vi "ImageColorRgbaU32ToArray.vi"(8 "error in":errorcluster, 10 "Optional Rectangle":T2, 11 "Image Reference In":T3) -> (0 "error out":errorcluster, 2 "Pixel":T1[][](array[typedef]), 3 "Image Reference Out":T3)   [LabVIEW 2020, in "OpenLvVision_Image.lvlib" / "DataAccess.lvlib"]
doc: "Copies the pixel into an 2D array without an border."
uses:
  DataAccess.lvlib
  Management/TypeDef/Image.ctl
  TypeDef/RectangleI32.ctl
  TypeDef/RgbaU32.ctl
  TypeDef/StepSizes.ctl
  Management/Management.lvlib
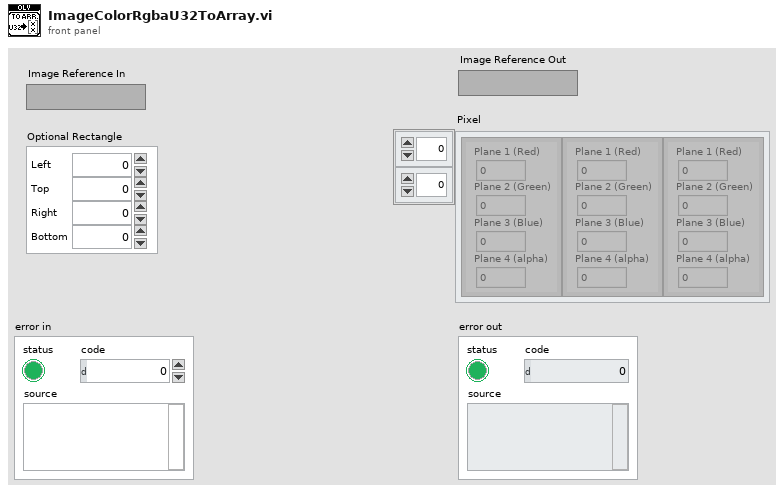
[diagram p1: front panel]
types:
  T1 = typedef "OpenLvVision_Image.lvlib/DataAccess.lvlib/RgbaU32.ctl" = cluster{"Plane 1 (Red)":u8, "Plane 2 (Green)":u8, "Plane 3 (Blue)":u8, "Plane 4 (alpha)":u8}
  T2 = typedef "OpenLvVision_Image.lvlib/DataAccess.lvlib/RectangleI32.ctl" = cluster{"Left":i32, "Top":i32, "Right":i32, "Bottom":i32}
  T3 = typedef "OpenLvVision_Image.lvlib/Management.lvlib/Image.ctl" = refnum<image>
  T4 = typedef "OpenLvVision_Image.lvlib/DataAccess.lvlib/StepSizes.ctl" = cluster{"X Step Size":u32, "Y Step Size":u32}
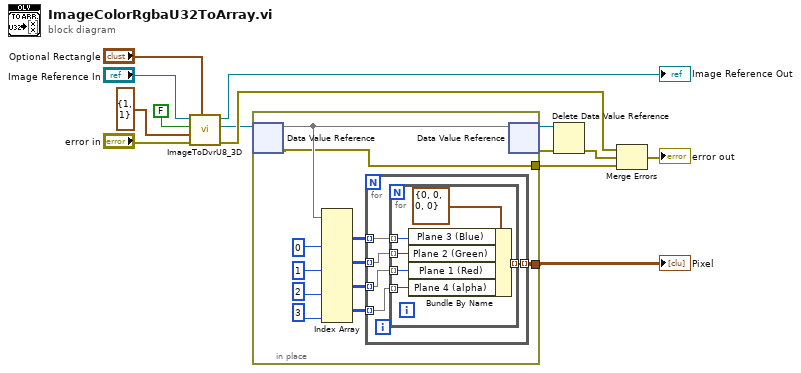
[diagram p0: block diagram]
diagram:
  n1 = call "ImageToDvrU8_3D.vi"("Optional Rectangle"="Optional Rectangle", "error in"="error in", "Step Sizes"=T4 {"X Step Size"=1, "Y Step Size"=1}, "Include Border"=FALSE, "Image Reference In"="Image Reference In") -> ("error out"=w5:errorcluster, "EDVR 3D U8"=w4:refnum<data-value>, "Image Reference Out"=→"Image Reference Out":T3)  [unwired: 3 in, 1 out]
  n2 = in-place {
    in-place-border: [w16] -> w1
    in-place-border: [w15] -> w2
    n3 = in-place-dvr #1(w4) -> (w25:u8[][][], w15:errorcluster)
    n4 = Index Array(array=w25, index (dim 2) #1=0, index (dim 2) #2=1, index (dim 2) #3=2, index (dim 2) #4=3) -> (element #1=w20:u8[][], element #2=w19:u8[][], element #3=w18:u8[][], element #4=w17:u8[][])  [unwired: 8 in]
    n5 = for {
      tunnel: w20 -> [w30] mode=indexing
      tunnel: w19 -> [w29] mode=indexing
      tunnel: w18 -> [w28] mode=indexing
      tunnel: w17 -> [w27] mode=indexing
      tunnel: [w26] -> w16 mode=indexing
      n6 = for {
        tunnel: w30 -> [w35] mode=indexing
        tunnel: w29 -> [w34] mode=indexing
        tunnel: w28 -> [w33] mode=indexing
        tunnel: w27 -> [w32] mode=indexing
        tunnel: [w31] -> w26 mode=indexing
        n7 = Bundle By Name(cluster=T1 {"Plane 1 (Red)"=0, "Plane 2 (Green)"=0, "Plane 3 (Blue)"=0, "Plane 4 (alpha)"=0} ("Color (U32)"), "Plane 3 (Blue)"=w35, "Plane 2 (Green)"=w34, "Plane 1 (Red)"=w33, "Plane 4 (alpha)"=w32) -> (w31:T1)
      }
    }
    n8 = in-place-dvr #1(w25) -> (w7:refnum<data-value>, w8:errorcluster)
  }
  "Pixel" <- w1
  n9 = Delete Data Value Reference(data value reference=w7, error in=w8) -> (error out=w3:errorcluster)  [unwired: 1 out]
  n10 = Merge Errors(w5, w3, w2) -> (→"error out":errorcluster)
